vi "Simulation Call Statechart.vi"(4 "operation":T6, 8 "error in":errorcluster, 10 "Multi Bot Sensors":T1[](array[typedef]) {"Kobuki Sensors"."Charger Source" items=["DISCHARGING"=0, "DOCKING_CHARGED"=2, "DOCKING_CHARGING"=6, "ADAPTER_CHARGED"=18, "ADAPTER_CHARGING"=22]; "accelerometer"."z axis (g)" format="%.3f"; "accelerometer"."y axis (g)" format="%.3f"; "accelerometer"."x axis (g)" format="%.3f"}, 11 "simulator":T10={"configuration"={"maxTime"=5.0, "enableVisualization"=TRUE, "Environment Definition"=path "iRobot Navigation State Machine.vi", "Record Location"=path "Simulation Record.xml", "autograde?"=TRUE, "interactive?"=FALSE, "Feedback Mode"=enum."debug navigation", "Robot State Charts"=[path "C:/Users/blueuser/Desktop/Robo Sim Berkley/cpsgrader-release-0.4/Simulators/EECS149lab/src/LabVIEW/statechart/Simulation Statechart.vi"], "statechart"=path "C:/Users/blueuser/Desktop/Robo Sim Berkley/cpsgrader-release-0.4/Simulators/EECS149lab/src/LabVIEW/statechart/Simulation Statechart.vi"}, "Statechart\ndisplay"=refnum, "first step?"=FALSE, "Robots Simulation Statecharts"=[], "Robots"=[]}) -> (0 "error out":errorcluster, 2 "trace element":T7 {"sensors"."Kobuki Sensors"."Charger Source" items=["DISCHARGING"=0, "DOCKING_CHARGED"=2, "DOCKING_CHARGING"=6, "ADAPTER_CHARGED"=18, "ADAPTER_CHARGING"=22]; "sensors"."accelerometer"."z axis (g)" format="%.3f"; "sensors"."accelerometer"."y axis (g)" format="%.3f"; "sensors"."accelerometer"."x axis (g)" format="%.3f"}, 3 "simulator":T10={"configuration"={"maxTime"=5.0, "enableVisualization"=TRUE, "Environment Definition"=path "iRobot Navigation State Machine.vi", "Record Location"=path "Simulation Record.xml", "autograde?"=TRUE, "interactive?"=FALSE, "Feedback Mode"=enum."debug navigation", "Robot State Charts"=[path "C:/Users/blueuser/Desktop/Robo Sim Berkley/cpsgrader-release-0.4/Simulators/EECS149lab/src/LabVIEW/statechart/Simulation Statechart.vi"], "statechart"=path "C:/Users/blueuser/Desktop/Robo Sim Berkley/cpsgrader-release-0.4/Simulators/EECS149lab/src/LabVIEW/statechart/Simulation Statechart.vi"}, "Statechart\ndisplay"=refnum, "first step?"=FALSE, "Robots Simulation Statecharts"=[], "Robots"=[]})   [LabVIEW 2015]
uses:
  Simulator.ctl
  CyberSim interface/Simulation Configuration.ctl
  autograder/feedbackMode.ctl
  Multi Bot Code/RobotData.ctl
  <instrlib>/DC Motor Controller/HAIOL/DC Motor Controller.lvclass
  Simulation Trace Element.ctl
  shared/Sensors.ctl
  shared/Accelerometer.ctl
  Kobuki/KobukiSensors.ctl
  Kobuki/Kobuki Bumps and WheelDrops.ctl
  Kobuki/Kobuki Buttons.ctl
  Simulated Position.ctl
  Simulated Orientation.ctl
  Simulation Call Statechart Operation.ctl
  Simulation Statechart Type.ctl
  Simulation Trace Operation.ctl
panel:
  # "Electrical: charging, battery, OI mode"
  # "Sensors: bump, cliff, button, wheel drop"
  # "Motors:"
  # "Inertia"
  # "Electrical: charging, battery, OI mode"
  # "Sensors: bump, cliff, button, wheel drop"
  # "Motors:"
  # "Inertia"
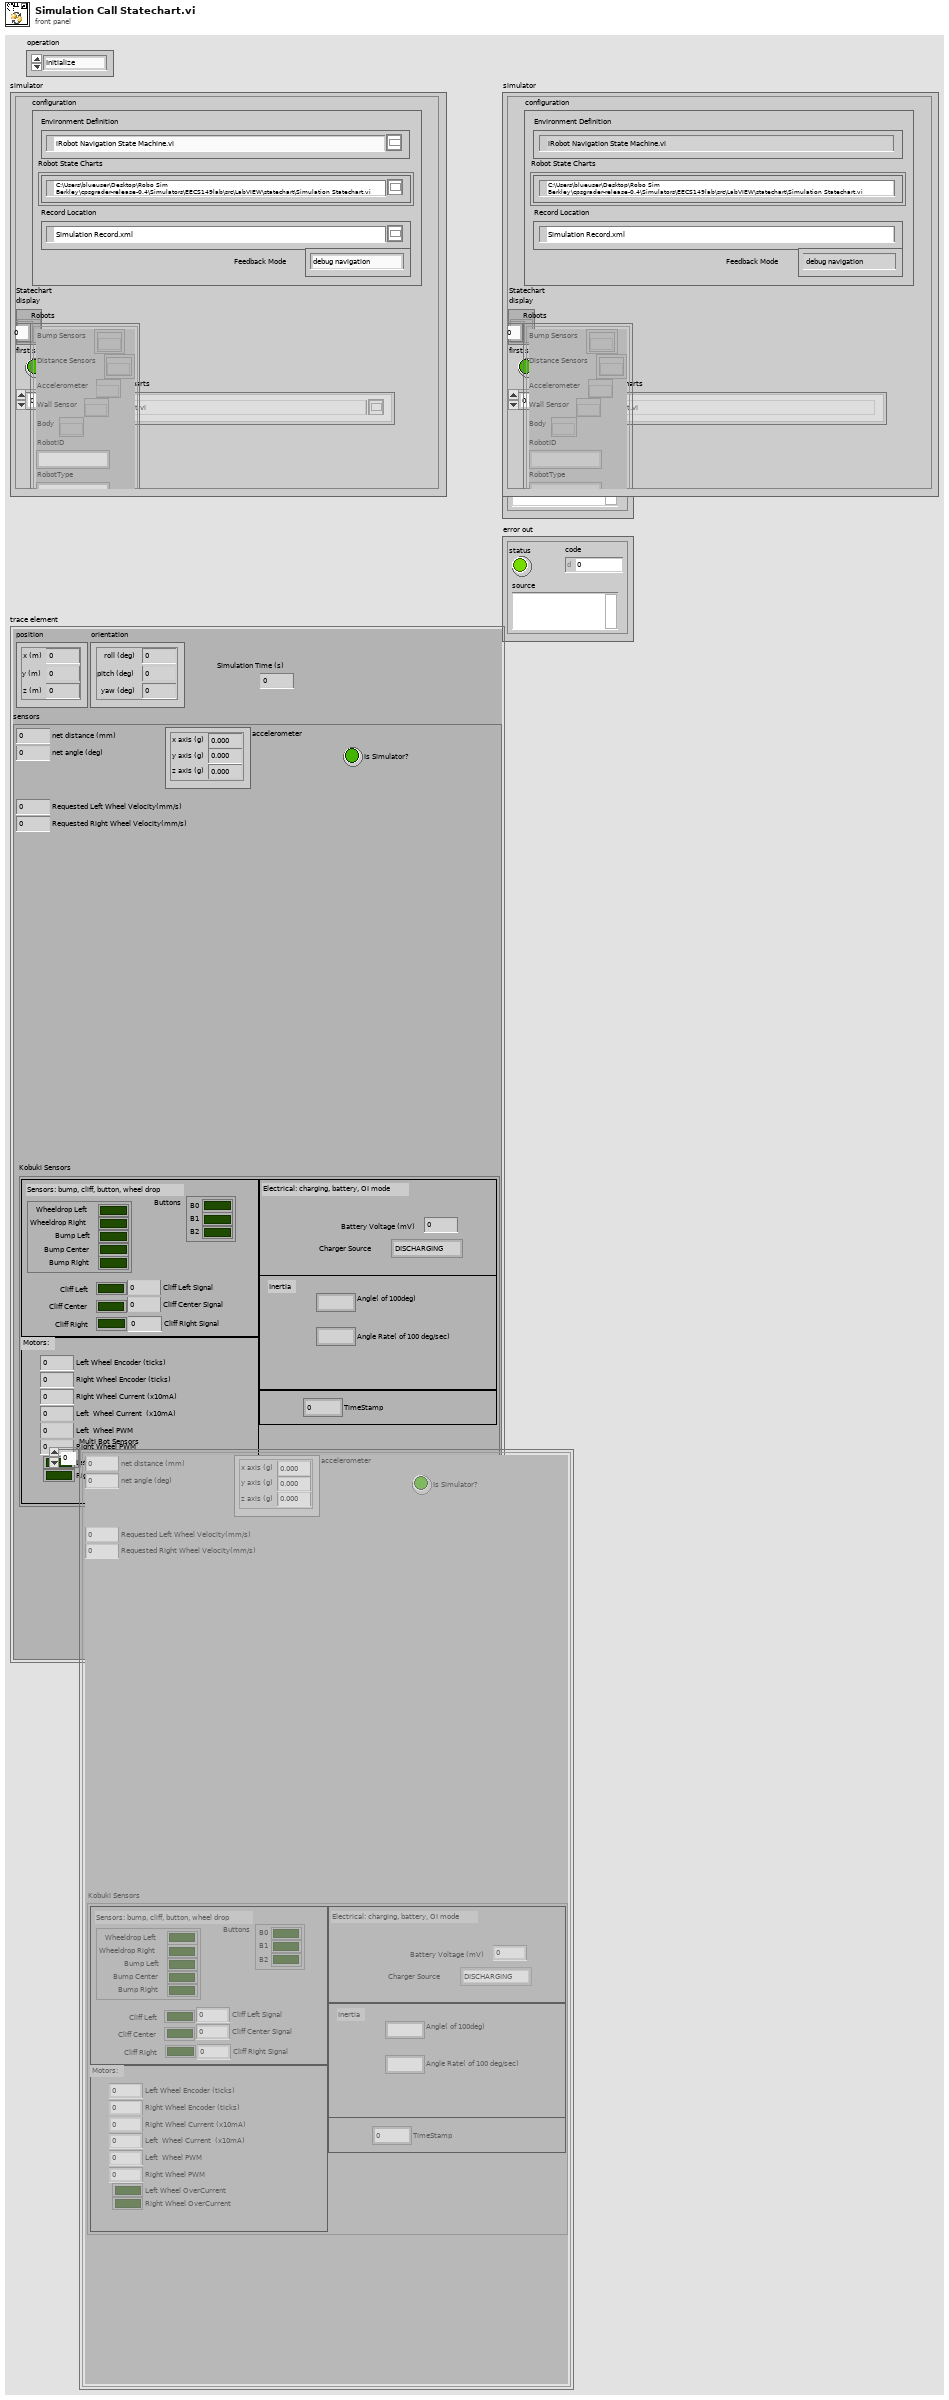
[diagram p1: front panel]
types:
  T1 = typedef "Sensors.ctl" = cluster{"net distance (mm)":i32, "net angle (deg)":i32, "accelerometer":T2, "Is Simulator?":bool, "Kobuki Sensors":T3, "Requested Left Wheel Velocity(mm/s)":i32, "Requested Right Wheel Velocity(mm/s)":i32}
  T2 = typedef "Accelerometer.ctl" = cluster{"x axis (g)":dbl, "y axis (g)":dbl, "z axis (g)":dbl}
  T3 = typedef "KobukiSensors.ctl" = cluster{"Bumps + Wheel Drops":T4, "Cliff Left":bool, "Cliff Center":bool, "Cliff Right":bool, "Cliff Left Signal":u16, "Cliff Center Signal":u16, "Cliff Right Signal":u16, "Buttons":T5, "Left Wheel Encoder (ticks)":u16, "Right Wheel Encoder (ticks) ":u16, "Left  Wheel PWM":i8, "Right Wheel PWM":i8, "Left Wheel OverCurrent":bool, "Right Wheel OverCurrent ":bool, "Right Wheel Current (x10mA)":i16, "Left  Wheel Current  (x10mA)":i16, "TimeStamp":u16, "Battery Voltage (mV)":i16, "Angle( of 100deg)":i16, "Angle Rate( of 100 deg/sec)":i16, "Charger Source ":i8}
  T4 = typedef "Kobuki Bumps and WheelDrops.ctl" = cluster{"Wheeldrop Left":bool, "Wheeldrop Right":bool, "Bump Left":bool, "Bump Center":bool, "Bump Right":bool}
  T5 = typedef "Kobuki Buttons.ctl" = cluster{"B0":bool, "B1":bool, "B2":bool}
  T6 = typedef "Simulation Call Statechart Operation.ctl" = enum16{"Initialize", "Call Statechart", "Finalize"}
  T7 = typedef "Simulation Trace Element.ctl" = cluster{"sensors":T1, "position":T8, "orientation":T9, "Simulation Time (s)":sgl}
  T8 = typedef "Simulated Position.ctl" = cluster{"x (m)":sgl, "y (m)":sgl, "z (m)":sgl}
  T9 = typedef "Simulated Orientation.ctl" = cluster{"roll (deg)":sgl, "pitch (deg)":sgl, "yaw (deg)":sgl}
  T10 = typedef "Simulator.ctl" = cluster{"configuration":T11, "Statechart\ndisplay":refnum<vi>, "first step?":bool, "Robots Simulation Statecharts":path[], "Robots":T13[]}
  T11 = typedef "Simulation Configuration.ctl" = cluster{"maxTime":sgl, "enableVisualization":bool, "Environment Definition":path, "Record Location":path, "autograde?":bool, "interactive?":bool, "Feedback Mode":T12, "Robot State Charts":path[], "statechart":path}
  T12 = typedef "feedbackMode.ctl" = enum32{"debug navigation", "debug hill climb", "autograde navigation", "autograde hill climb"}
  T13 = typedef "RobotData.ctl" = cluster{"Bump Sensors":refnum<k20>[], "Distance Sensors":refnum<k20>[], "Accelerometer":refnum<k20>, "Wall Sensor":refnum<k20>, "Body":refnum<k20>, "RobotID":string, "RobotType":string, "Left Motor":refnum<class "DC Motor Controller.lvclass">, "Right Motor":refnum<class "DC Motor Controller.lvclass">}
  T14 = typedef "Simulation Statechart Type.ctl" = enum16{"Unknown", "LabVIEW VI", "DLL"}
  T15 = typedef "Simulation Trace Operation.ctl" = enum16{"Initialize", "Record Trace Element", "Get Trace"}
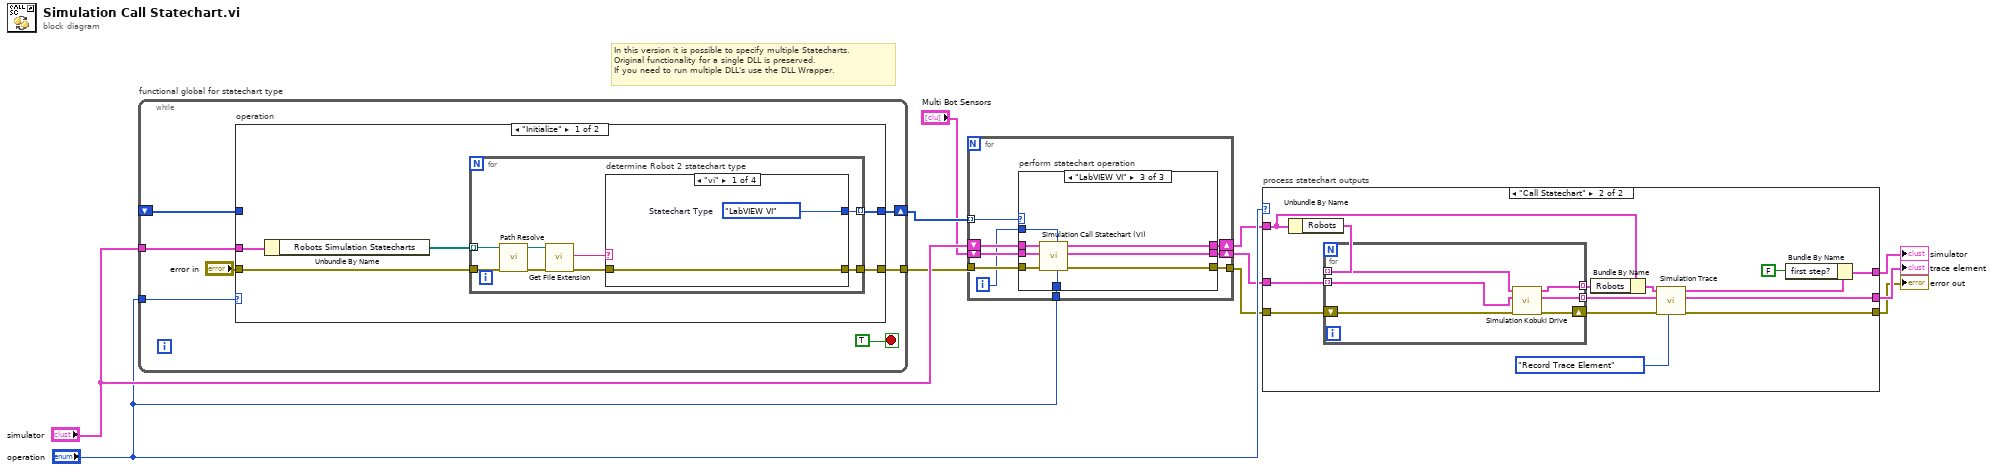
[diagram p0: block diagram]
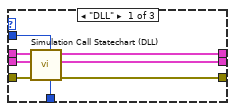
[diagram p2: hidden frame]
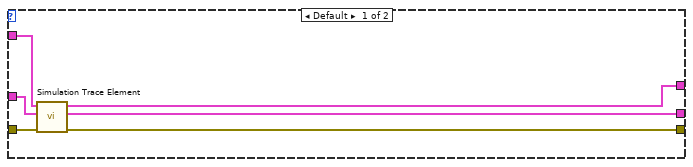
[diagram p4: hidden frame]
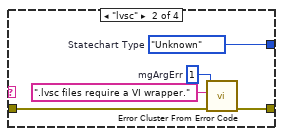
[diagram p5: hidden frame]
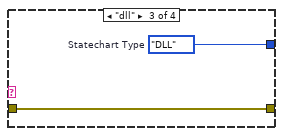
[diagram p6: hidden frame]
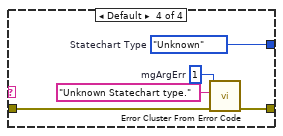
[diagram p7: hidden frame]
diagram:
  # "In this version it is possible to specify multiple Statecharts. \nOriginal functionality for a single DLL is preserved.\nIf you need to run multiple DLL's use the DLL Wrapper."
  n1 = while "functional global for statechart type" {
    tunnel: "operation" -> [w15]
    tunnel: "simulator" -> [w18]
    shift-right: [w14] -> w6
    shift-left: _ -> [w13]
    tunnel: [w12] -> w3
    stop <- TRUE stop-if-true
    n2 = case "operation" shown="\"Initialize\"" w15 {
      tunnel: w18 -> [w23 _]
      tunnel: "error in" -> [w20 w46]
      tunnel: [w21 w47] -> w14
      tunnel: w13 -> [_ w47]
      tunnel: [w19 w46] -> w12
      frame "Initialize" {
        n3 = Unbundle By Name(w23) -> ("Robots Simulation Statecharts"=w22:path[])
        n4 = for {
          tunnel: w22 -> [w27] mode=indexing
          tunnel: w20 -> [w26]
          tunnel: [w25] -> w21 mode=indexing
          tunnel: [w24] -> w19
          n5 = call "Path Resolve.vi"("Error In"=w26, "absolute or relative path"=w27) -> ("Error Out"=w30:errorcluster, "resolved path"=w31:path)  [unwired: 8 in]
          n6 = call <vilib>:"Get File Extension.vi"("error in (no error)"=w30, "file"=w31) -> ("error out"=w29:errorcluster, "lowercase file extension"=w28:string)  [unwired: 5 in, 3 out]
          n7 = case "determine Robot 2 statechart type" shown="\"vi\"" w28 {
            tunnel: w29 -> [w33 w36 w39 w43]
            tunnel: [w33 w35 w39 w42] -> w24
            tunnel: [w32 w34 w40 w41] -> w25
            frame "vi" {
              w32 = Simulation_Statechart_Type."LabVIEW VI"  # Statechart Type
            }
            frame "lvsc" {
              w34 = Simulation_Statechart_Type."Unknown"  # Statechart Type
              w37 = 1  # mgArgErr
              n8 = call <vilib>:"Error Cluster From Error Code.vi"("error in (no error)"=w36, "error message (\"\")"=".lvsc files require a VI wrapper." ("error message (\"\")"), "error code (0)"=w37) -> ("error out"=w35:errorcluster)  [unwired: 6 in]
            }
            frame "dll" {
              w40 = Simulation_Statechart_Type."DLL"  # Statechart Type
            }
            frame Default {
              w41 = Simulation_Statechart_Type."Unknown"  # Statechart Type
              w44 = 1  # mgArgErr
              n9 = call <vilib>:"Error Cluster From Error Code.vi"("error in (no error)"=w43, "error message (\"\")"="Unknown Statechart type." ("error message (\"\")"), "error code (0)"=w44) -> ("error out"=w42:errorcluster)  [unwired: 6 in]
            }
          }
        }
      }
      frame Default {
      }
    }
  }
  n10 = for {
    tunnel: w3 -> [w56]
    tunnel: "operation" -> [w54]
    tunnel: w6 -> [w53] mode=indexing
    tunnel: [w50] -> w1
    shift-right: [w52] -> w5
    shift-left: "Multi Bot Sensors" -> [w49]
    shift-right: [w51] -> w2
    shift-left: "simulator" -> [w55]
    i -> [w48]
    n11 = case "perform statechart operation" shown="\"LabVIEW VI\"" w53 {
      tunnel: w56 -> [w62 w65 w73]
      tunnel: w55 -> [w64 w67 w75]
      tunnel: w54 -> [w61 _ w69]
      tunnel: w49 -> [w63 w66 w74]
      tunnel: [w60 w67 w72] -> w51
      tunnel: [w59 w66 w71] -> w52
      tunnel: [w58 w65 w70] -> w50
      tunnel: w48 -> [w57 _ w68]
      frame "DLL" {
        n12 = call "Simulation Call Statechart (DLL).vi"("operation"=w61, "Robot Index"=w57, "error in (no error)"=w62, "Array Sensors In"=w63, "simulator"=w64) -> ("error out"=w58:errorcluster, "Array Sensors Out"=w59:T1[], "simulator"=w60:T10)  [unwired: 4 in]
      }
      frame "Unknown", Default {
      }
      frame "LabVIEW VI" {
        n13 = call "Simulation Call Statechart (VI).vi"("operation"=w69, "Robot Index"=w68, "error in"=w73, "Array of Sensors In"=w74, "simulator"=w75) -> ("error out"=w70:errorcluster, "Array of Sensors Out"=w71:T1[], "simulator"=w72:T10)  [unwired: 4 in]
      }
    }
  }
  n14 = case "process statechart outputs" shown="\"Call Statechart\"" "operation" {
    tunnel: w2 -> [w81 w89]
    tunnel: w1 -> [w77 w88]
    tunnel: [w80 w92] -> w11
    tunnel: [w79 w91] -> w10
    tunnel: [w78 w90] -> w9
    tunnel: w5 -> [w76 w85]
    frame Default {
      n15 = call "Simulation Trace Element.vi"("error in (no error)"=w77, "Sensors Array"=w76, "simulator"=w81) -> ("error out"=w78:errorcluster, "trace element"=w79:T7, "simulator"=w80:T10)  [unwired: 6 in]
    }
    frame "Call Statechart" {
      n16 = Unbundle By Name(w89) -> ("Robots"=w86:T13[])
      n17 = for {
        shift-right: [w100] -> w87
        shift-left: w88 -> [w101]
        tunnel: w86 -> [w99] mode=indexing
        tunnel: w85 -> [w96] mode=indexing
        tunnel: [w98] -> w84 mode=indexing
        tunnel: [w97] -> w82 mode=indexing
        n18 = call "Simulation Kobuki Drive.vi"("error in"=w101, "sensors"=w96, "Robot In"=w99) -> ("error out"=w100:errorcluster, "sensors"=w97:T1, "Robot Out"=w98:T13)  [unwired: 6 in]
      }
      n19 = Bundle By Name(cluster=w89, "Robots"=w84) -> (w83:T10)
      n20 = call "Simulation Trace.vi"("operation"=Simulation_Trace_Operation."Record Trace Element", "error in"=w87, "Sensors Array"=w82, "simulator"=w83) -> ("error out"=w90:errorcluster, "last trace element"=w91:T7, "simulator"=w93:T10)  [unwired: 4 in, 1 out]
      n21 = Bundle By Name(cluster=w93, "first step?"=FALSE ("init?")) -> (w92:T10)
    }
  }
  "error out" <- w9
  "simulator" <- w11
  "trace element" <- w10
